vi "Pump Status.vi"(8 "error in (no error)":errorcluster, 11 "Pump Calibration Config in":T1={"Settings"={"Cycle Period"=500.0, "Ismatech"={"VISA resource name"="", "Simulated?"=TRUE, "Pump Number"=1.0, "Reverse?"=FALSE}, "Masterflex"={"VISA resource name"="", "Simulated?"=TRUE, "Pump Number"=1.0, "Reverse?"=FALSE}, "Bronkhorst M13 Settings"={"VISA resource name"="", "Simulated?"=TRUE, "Smoothing Steps"=1}, "PID 2 Parameters"={"Input Device"=enum."Default", "Output Device"=enum."Default"}, "Tacmina Settings"={"Analog DAQ Task"="", "Digital DAQ Task"=""}, "KNF SIMDOS Settings"={"VISA resource name"="", "Simulated?"=TRUE}, "VICI M50 Settings"={"VISA resource name"="", "Pump ID"="", "Pump Head Vol"=0.0, "Reverse?"=FALSE, "Simulated?"=TRUE}, "FLOM Settings"={"VISA resource name"="", "Simulated?"=TRUE, "Pump Number"=0.0}, "Calibration Limits"={"Minimum (ml/min)"=0.0, "Maximum (ml/min)"=0.0, "Steps"=0.0}, "SSI PR Settings"={"VISA resource name"="", "Simulated?"=FALSE}, "Ismatech 4308 Settings"={"VISA resource name"="", "Pump Number"=1, "Channel Number"=0, "Simulated?"=TRUE, "Reverse?"=FALSE}, "Bronkhorst M14 Settings"={"VISA resource name"="", "Simulated?"=FALSE, "Smoothing Steps"=1}}, "Flowmeter Output"=0.0, "Density"=0.0, "FL Temp"=0.0, "Speed %"=0.0, "File Refnum"=refnum, "Pump On?"=enum."Not Initialized"} {"Settings"."Bronkhorst M14 Settings"."Smoothing Steps" min=1 step=1; "Settings"."Ismatech 4308 Settings"."Channel Number" min=0 max=3; "Settings"."Ismatech 4308 Settings"."Pump Number" min=1; "Settings"."Bronkhorst M13 Settings"."Smoothing Steps" min=1 step=1; "Settings"."Masterflex"."Pump Number" min=1.0 max=20.0 step=1.0; "Settings"."Ismatech"."Pump Number" min=1.0 max=20.0 step=1.0}) -> (0 "error out":errorcluster, 3 "Pump Calibration Config out":T1={"Settings"={"Cycle Period"=500.0, "Ismatech"={"VISA resource name"="", "Simulated?"=TRUE, "Pump Number"=1.0, "Reverse?"=FALSE}, "Masterflex"={"VISA resource name"="", "Simulated?"=TRUE, "Pump Number"=1.0, "Reverse?"=FALSE}, "Bronkhorst M13 Settings"={"VISA resource name"="", "Simulated?"=TRUE, "Smoothing Steps"=1}, "PID 2 Parameters"={"Input Device"=enum."Default", "Output Device"=enum."Default"}, "Tacmina Settings"={"Analog DAQ Task"="", "Digital DAQ Task"=""}, "KNF SIMDOS Settings"={"VISA resource name"="", "Simulated?"=TRUE}, "VICI M50 Settings"={"VISA resource name"="", "Pump ID"="", "Pump Head Vol"=0.0, "Reverse?"=FALSE, "Simulated?"=TRUE}, "FLOM Settings"={"VISA resource name"="", "Simulated?"=TRUE, "Pump Number"=0.0}, "Calibration Limits"={"Minimum (ml/min)"=0.0, "Maximum (ml/min)"=0.0, "Steps"=0.0}, "SSI PR Settings"={"VISA resource name"="", "Simulated?"=FALSE}, "Ismatech 4308 Settings"={"VISA resource name"="", "Pump Number"=1, "Channel Number"=0, "Simulated?"=TRUE, "Reverse?"=FALSE}, "Bronkhorst M14 Settings"={"VISA resource name"="", "Simulated?"=FALSE, "Smoothing Steps"=1}}, "Flowmeter Output"=0.0, "Density"=0.0, "FL Temp"=0.0, "Speed %"=0.0, "File Refnum"=refnum, "Pump On?"=enum."Not Initialized"} {"Settings"."Bronkhorst M14 Settings"."Smoothing Steps" min=1 step=1; "Settings"."Ismatech 4308 Settings"."Channel Number" min=0 max=3; "Settings"."Ismatech 4308 Settings"."Pump Number" min=1; "Settings"."Bronkhorst M13 Settings"."Smoothing Steps" min=1 step=1; "Settings"."Masterflex"."Pump Number" min=1.0 max=20.0 step=1.0; "Settings"."Ismatech"."Pump Number" min=1.0 max=20.0 step=1.0})   [LabVIEW 2018, in "Calibration.lvlib" / "Engine.lvlib"]
uses:
  Engine.lvlib
  Pump Calibration Config.ctl
  Pfizer Timed Seq/Software/Ismatec ISM 831C/Controls/Ismatech ISM831C Settings Cluster.ctl
  Pfizer Timed Seq/Software/Masterflex 7550-30/Controls/Settings Cluster.ctl
  Pfizer Timed Seq/Software/Bronkhorst M13 Flow Meter/Settings Cluster.ctl
  Pfizer Timed Seq/Software/Measure Instrument/PID Input Enum.ctl
  Pfizer Timed Seq/Software/Measure Instrument/PID 2 Output Enum.ctl
  Pfizer Timed Seq/Software/Tacmina QI/Tacmina QI DAQ Setting.ctl
  Pfizer Timed Seq/Software/KNF Pump/Settings Cluster plus SIMDOS.ctl
  Pfizer Timed Seq/Software/VICI M50 Party Mode/Settings Cluster.ctl
  Pfizer Timed Seq/Software/FLOM Pump/Settings Cluster.ctl
  Pfizer Timed Seq/Software/SSI PR Class/SSI PR or LD Settings Cluster.ctl
  Pfizer Timed Seq/Software/Ismatec 78001/Ismatec 4083.ctl
  Pfizer Timed Seq/Software/Bronkhorst M14 Flow Meter/Settings Cluster.ctl
  Pfizer Timed Seq/Software/Ismatec ISM 831C/Ismatec ISM 831C.lvlib
  Pfizer Timed Seq/Software/Masterflex 7550-30/Masterflex 7550-30.lvlib
  Pfizer Timed Seq/Software/VICI M50 Party Mode/VICI M6 M50 Party Mode.lvlib
  Pfizer Timed Seq/Software/Tacmina QI/Tacmina QI.lvlib
  Pfizer Timed Seq/Software/KNF Pump/KNF SIMDOS.lvlib
  Pfizer Timed Seq/Software/FLOM Pump/FLOM Pump.lvlib
  Pfizer Timed Seq/Software/SSI PR Class/SSI PR or LD Pump.lvlib
  Pfizer Timed Seq/Software/Ismatec 78001/Ismatec 4308.lvlib
  Pfizer Timed Seq/Software/Bronkhorst M13 Flow Meter/Bronkhorst M13 Flow Meter.lvlib
  Pfizer Timed Seq/Software/Calibration VIs/Calibration.lvlib
  Pfizer Timed Seq/Software/Bronkhorst M14 Flow Meter/Bronkhorst M14 Flow Meter.lvlib
panel:
  # "Output Instruments"
  # "Input Instruments"
  # "Output Instruments"
  # "Input Instruments"
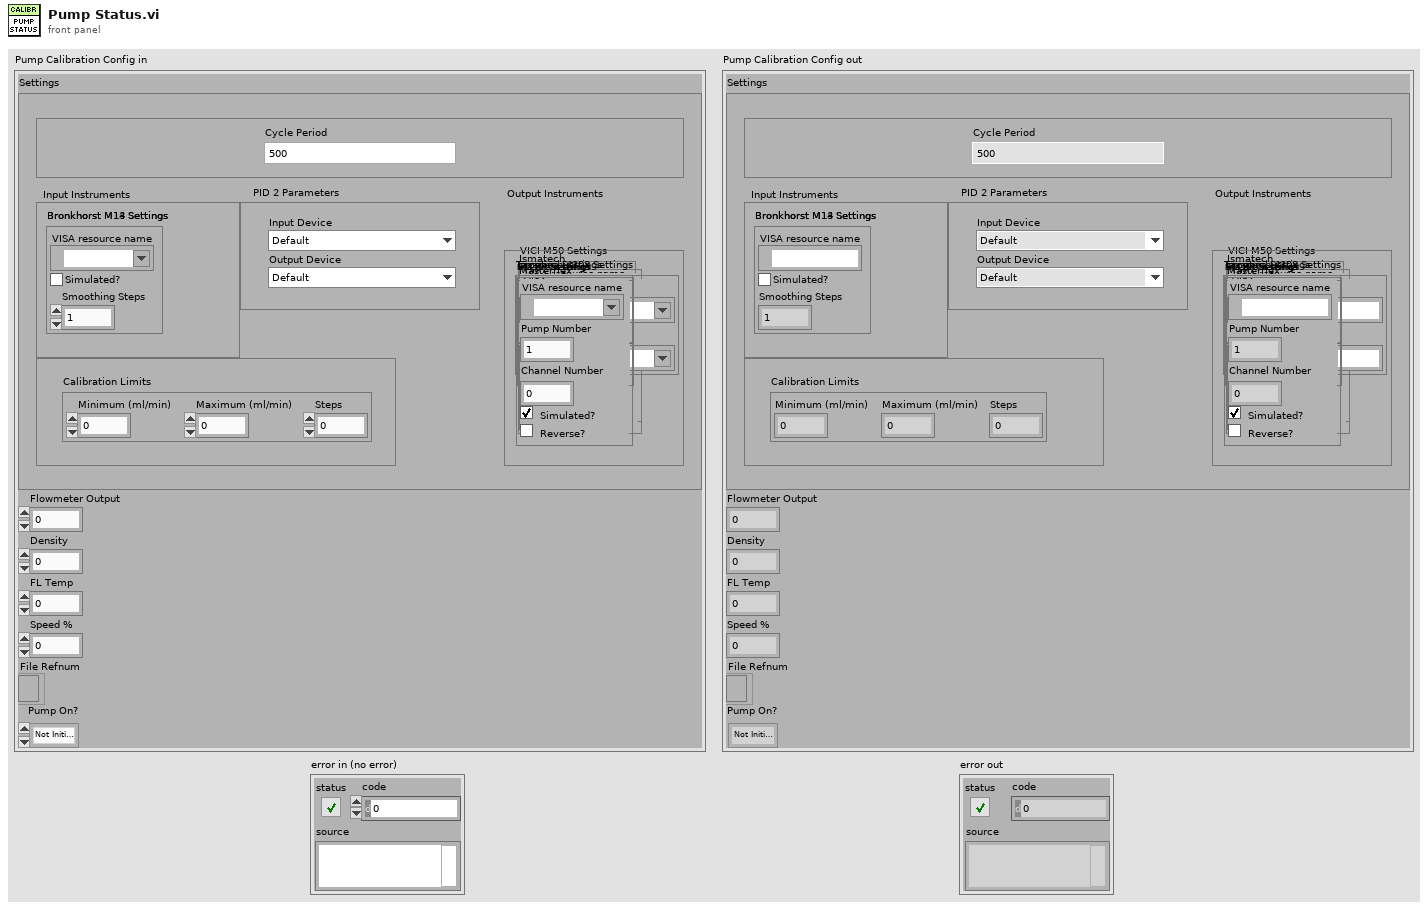
[diagram p1: front panel]
types:
  T1 = typedef "Calibration.lvlib/Pump Calibration Config.ctl" = cluster{"Settings":cluster{"Cycle Period":dbl, "Ismatech":T2, "Masterflex":T3, "Bronkhorst M13 Settings":T4, "PID 2 Parameters":cluster{"Input Device":T5, "Output Device":T6}, "Tacmina Settings":T7, "KNF SIMDOS Settings":T8, "VICI M50 Settings":T9, "FLOM Settings":T10, "Calibration Limits":cluster{"Minimum (ml/min)":dbl, "Maximum (ml/min)":dbl, "Steps":dbl}, "SSI PR Settings":T11, "Ismatech 4308 Settings":T12, "Bronkhorst M14 Settings":T13}, "Flowmeter Output":dbl, "Density":dbl, "FL Temp":dbl, "Speed %":dbl, "File Refnum":refnum<file>, "Pump On?":enum16{"Off", "On", "Not Initialized"}}
  T2 = typedef "Ismatec ISM 831C.lvlib/Ismatech ISM831C Settings Cluster.ctl" = cluster{"VISA resource name":refnum<visa-resource-name>, "Simulated?":bool, "Pump Number":dbl, "Reverse?":bool}
  T3 = typedef "Masterflex 7550-30.lvlib/Settings Cluster.ctl" = cluster{"VISA resource name":refnum<visa-resource-name>, "Simulated?":bool, "Pump Number":dbl, "Reverse?":bool}
  T4 = typedef "Bronkhorst M13 Flow Meter.lvlib/Settings Cluster.ctl" = cluster{"VISA resource name":refnum<visa-resource-name>, "Simulated?":bool, "Smoothing Steps":i32}
  T5 = typedef "PID Input Enum.ctl" = enum16{"Default", "Bronkhorst M13", "Bronkhorst M14", "Scale Rate of Change"}
  T6 = typedef "PID 2 Output Enum.ctl" = enum16{"Default", "Ismatec ISM 4308", "Ismatec ISM 831C", "Masterflex 7550-30", "VICI M6", "VICI M50", "Tacmina QI", "KNF SIMDOS", "ASIA Type C", "FLOM UI-22-11", "SSI PR/LD", "SSI P40", "Masterflex 75211-70"}
  T7 = typedef "Tacmina QI.lvlib/Tacmina QI DAQ Setting.ctl" = cluster{"Analog DAQ Task":refnum<k21>, "Digital DAQ Task":refnum<k21>}
  T8 = typedef "KNF SIMDOS.lvlib/Settings Cluster plus SIMDOS.ctl" = cluster{"VISA resource name":refnum<visa-resource-name>, "Simulated?":bool}
  T9 = typedef "VICI M6 M50 Party Mode.lvlib/Settings Cluster.ctl" = cluster{"VISA resource name":refnum<visa-resource-name>, "Pump ID":string, "Pump Head Vol":dbl, "Reverse?":bool, "Simulated?":bool}
  T10 = typedef "FLOM Pump.lvlib/Settings Cluster.ctl" = cluster{"VISA resource name":refnum<visa-resource-name>, "Simulated?":bool, "Pump Number":dbl}
  T11 = typedef "SSI PR or LD Pump.lvlib/SSI PR or LD Settings Cluster.ctl" = cluster{"VISA resource name":refnum<visa-resource-name>, "Simulated?":bool}
  T12 = typedef "Ismatec 4308.lvlib/Ismatec 4083.ctl" = cluster{"VISA resource name":refnum<visa-resource-name>, "Pump Number":i16, "Channel Number":i16, "Simulated?":bool, "Reverse?":bool}
  T13 = typedef "Bronkhorst M14 Flow Meter.lvlib/Settings Cluster.ctl" = cluster{"VISA resource name":refnum<visa-resource-name>, "Simulated?":bool, "Smoothing Steps":i32}
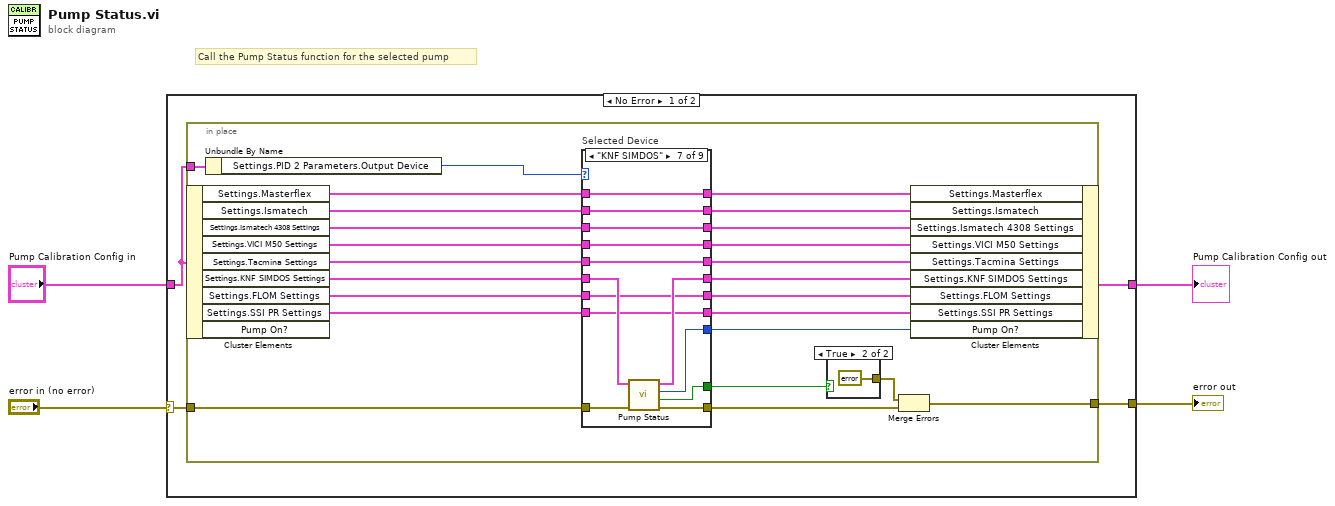
[diagram p0: block diagram]
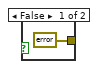
[diagram p2: hidden frame]
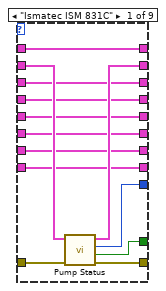
[diagram p3: hidden frame]
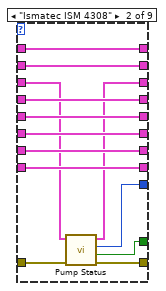
[diagram p4: hidden frame]
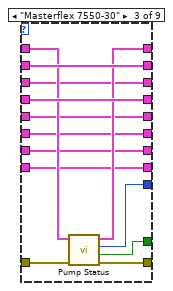
[diagram p5: hidden frame]
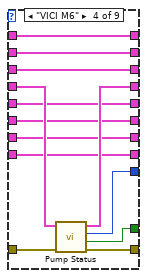
[diagram p6: hidden frame]
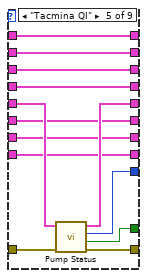
[diagram p7: hidden frame]
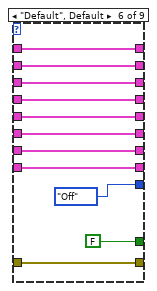
[diagram p8: hidden frame]
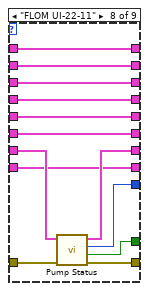
[diagram p9: hidden frame]
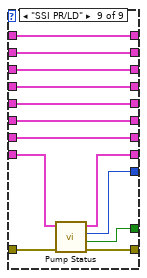
[diagram p10: hidden frame]
diagram:
  # "Call the Pump Status function for the selected pump"
  n1 = case shown="No Error" "error in (no error)" {
    selector: "error in (no error)" -> [w8 w151]
    tunnel: [w5 w151] -> w3
    tunnel: "Pump Calibration Config in" -> [w7 w150]
    tunnel: [w6 w150] -> w1
    frame No Error {
      n2 = in-place {
        in-place-border: w7 -> [w32]
        in-place-border: w8 -> [w31]
        in-place-border: [w13] -> w5
        n3 = in-place-cluster #1(w7) -> ("Settings.Masterflex"=w28:T3, "Settings.Ismatech"=w27:T2, "Settings.Ismatech 4308 Settings"=w9:T12, "Settings.VICI M50 Settings"=w26:T9, "Settings.Tacmina Settings"=w25:T7, "Settings.KNF SIMDOS Settings"=w24:T8, "Settings.FLOM Settings"=w23:T10, "Settings.SSI PR Settings"=w22:T11)  [unwired: 1 out]
        n4 = Unbundle By Name(w32) -> ("Settings.PID 2 Parameters.Output Device"=w30:T6)
        n5 = case "Selected Device" shown="\"KNF SIMDOS\"" w30 {
          tunnel: w28 -> [w47 w60 w69 w85 w99 w110 w123 w136 w138]
          tunnel: [w47 w60 w70 w85 w99 w110 w123 w136 w138] -> w21
          tunnel: w27 -> [w45 w54 w73 w86 w98 w109 w122 w135 w149]
          tunnel: [w46 w51 w71 w82 w95 w103 w119 w131 w143] -> w11
          tunnel: w31 -> [w37 w50 w63 w76 w89 w103 w113 w126 w144]
          tunnel: [w44 w54 w73 w86 w98 w109 w122 w135 w149] -> w20
          tunnel: w26 -> [w42 w58 w72 w83 w97 w108 w121 w134 w148]
          tunnel: [w42 w58 w72 w84 w97 w108 w121 w134 w148] -> w19
          tunnel: w25 -> [w43 w59 w68 w81 w96 w107 w120 w133 w147]
          tunnel: [w43 w59 w68 w81 w94 w107 w120 w133 w147] -> w18
          tunnel: [w41 w57 w67 w80 w93 w106 w118 w132 w146] -> w17
          tunnel: w24 -> [w41 w57 w67 w80 w93 w106 w117 w132 w146]
          tunnel: [w40 w53 w66 w79 w92 enum16{"Off", "On", "Not Initialized"}."Off" ("Pump On?") w116 w128 w141] -> w14
          tunnel: [w39 w56 w65 w78 w91 w104 w115 w130 w145] -> w16
          tunnel: w23 -> [w39 w56 w65 w78 w91 w104 w115 w129 w145]
          tunnel: [w38 w52 w64 w77 w90 FALSE ("Connection Error") w114 w127 w142] -> w29
          tunnel: w22 -> [w36 w55 w62 w75 w88 w101 w112 w125 w140]
          tunnel: [w36 w55 w62 w75 w88 w101 w112 w125 w139] -> w15
          tunnel: [w35 w48 w61 w74 w87 w100 w111 w124 w137] -> w10
          tunnel: w9 -> [w35 w49 w61 w74 w87 w100 w111 w124 w137]
          frame "Ismatec ISM 831C" {
            n6 = call "Pump Status.vi"("error in (no error)"=w37, "Ismatech Settings In"=w45) -> ("error out"=w46:errorcluster, "Connection Error"=w38:bool, "Pump On?"=w40:enum16{"Off", "On", "Not Initialized"}, "Ismatech Settings Out"=w44:T2)  [unwired: 6 in]
          }
          frame "Ismatec ISM 4308" {
            n7 = call "Pump Status.vi"("error in (no error)"=w50, "Ismatech 3 Channel Settings In"=w49) -> ("error out"=w51:errorcluster, "Connection Error"=w52:bool, "Pump On?"=w53:enum16{"Off", "On", "Not Initialized"}, "Ismatech 3 Channel Settings Out"=w48:T12)  [unwired: 5 in, 1 out]
          }
          frame "Masterflex 7550-30" {
            n8 = call "Pump Status.vi"("error in (no error)"=w63, "Masterflex Settings in"=w69) -> ("error out"=w71:errorcluster, "Connection Error"=w64:bool, "Pump On?"=w66:enum16{"Off", "On", "Not Initialized"}, "Masterflex Settings out"=w70:T3)  [unwired: 6 in]
          }
          frame "VICI M6" {
            n9 = call "Pump Status.vi"("error in (no error)"=w76, "VICI Settings In"=w83) -> ("error out"=w82:errorcluster, "Connection Error"=w77:bool, "Pump On?"=w79:enum16{"Off", "On", "Not Initialized"}, "VICI Settings Out"=w84:T9)  [unwired: 6 in]
          }
          frame "Tacmina QI" {
            n10 = call "Pump Status.vi"("error in"=w89, "Tacmina Settings in"=w96) -> ("error out"=w95:errorcluster, "Connection Error"=w90:bool, "Pump On?"=w92:enum16{"Off", "On", "Not Initialized"}, "Tacmina Settings out"=w94:T7)  [unwired: 6 in]
          }
          frame "Default", Default {
          }
          frame "KNF SIMDOS" {
            n11 = call "Pump Status.vi"("error in (no error)"=w113, "KNF Settings In"=w117) -> ("error out"=w119:errorcluster, "Connection Error"=w114:bool, "Pump On?"=w116:enum16{"Off", "On", "Not Initialized"}, "KNF Settings Out"=w118:T8)  [unwired: 6 in]
          }
          frame "FLOM UI-22-11" {
            n12 = call "Pump Status.vi"("error in (no error)"=w126, "FLOM Settings In"=w129) -> ("error out"=w131:errorcluster, "Connection Error"=w127:bool, "Pump On?"=w128:enum16{"Off", "On", "Not Initialized"}, "FLOM Settings Out"=w130:T10)  [unwired: 4 in, 2 out]
          }
          frame "SSI PR/LD" {
            n13 = call "Pump Status.vi"("error in (no error)"=w144, "SSI PR Settings"=w140) -> ("error out"=w143:errorcluster, "Connection Error"=w142:bool, "Pump On?"=w141:enum16{"Off", "On", "Not Initialized"}, "SSI PR Settings"=w139:T11)  [unwired: 4 in, 2 out]
          }
        }
        n14 = case shown="True" w29 {
          tunnel: [errorcluster {"status"=FALSE, "code"=0, "source"=""} ("error constant") errorcluster {"status"=TRUE, "code"=3, "source"="Pump Connection Error"} ("error constant")] -> w12
          frame False {
          }
          frame True {
          }
        }
        n15 = Merge Errors(w12, w11) -> (w13:errorcluster)
        n16 = in-place-cluster #1("Settings.Masterflex"=w21, "Settings.Ismatech"=w20, "Settings.Ismatech 4308 Settings"=w10, "Settings.VICI M50 Settings"=w19, "Settings.Tacmina Settings"=w18, "Settings.KNF SIMDOS Settings"=w17, "Settings.FLOM Settings"=w16, "Settings.SSI PR Settings"=w15, "Pump On?"=w14) -> (w6:T1)
      }
    }
    frame Error {
    }
  }
  "error out" <- w3
  "Pump Calibration Config out" <- w1
